vi "New.vi"(11 "VISA resource name":refnum<visa-resource-name>) -> (0 "error out":errorcluster, 3 "Motor out":refnum<class "Motor.lvclass">)   [LabVIEW 2019, in "Motor.lvclass"]
uses:
  Motor.lvclass
  Motor.lvclass/Motor.ctl
  Motor Serial class/Serial.lvclass
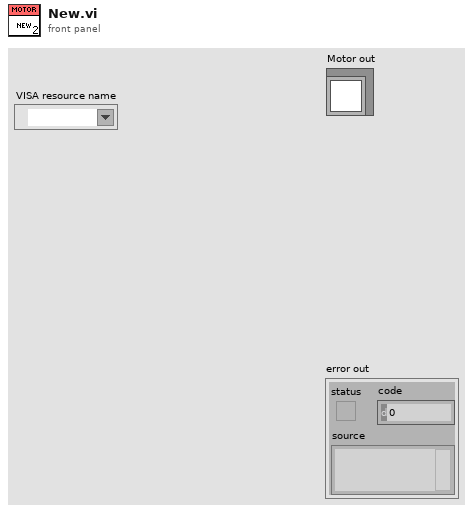
[diagram p1: front panel]
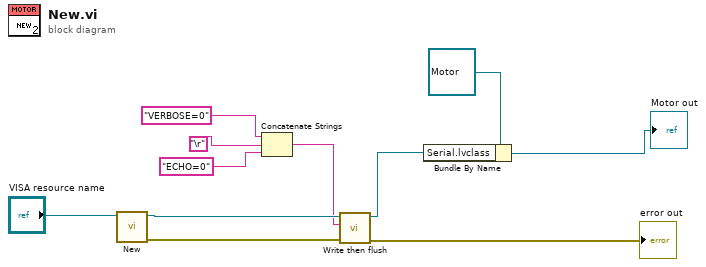
[diagram p0: block diagram]
diagram:
  n1 = call "New.vi"("VISA resource name"="VISA resource name") -> ("error out"=w6:errorcluster, "Motor_Serial out"=w7:refnum<class "Serial.lvclass">)  [unwired: 9 in]
  n2 = Concatenate Strings("VERBOSE=0" ("string"), "\r", "ECHO=0" ("string")) -> (w5:string)
  n3 = call "Write then flush.vi"("error in (no error)"=w6, "TX Data"=w5, "Motor_Serial in"=w7) -> ("error out"=→"error out":errorcluster, "Motor_Serial out"=w4:refnum<class "Serial.lvclass">)  [unwired: 7 in]
  n4 = Bundle By Name(cluster=refnum<class "Motor.lvclass"> refnum ("Motor.lvclass"), "Serial.lvclass"=w4) -> (→"Motor out":refnum<class "Motor.lvclass">)
